vi "Lookup Form Field.vi"   [LabVIEW 2020]
uses:
  lv-http-util/HTTP Utils/Request/Request.lvclass
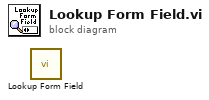
[diagram p0: block diagram]
diagram:
  n1 = call "Lookup Form Field.vi"() -> ()  [unwired: 8 in, 4 out]
